vi "concentration percent.vi"(10 "Type Conentration":enum32{"Item 0", "Item 1"}(radio), 11 "Concentration In":T1) -> (3 "Concentration Out":T1)   [LabVIEW 2023]
uses:
  control/Concentrations.ctl
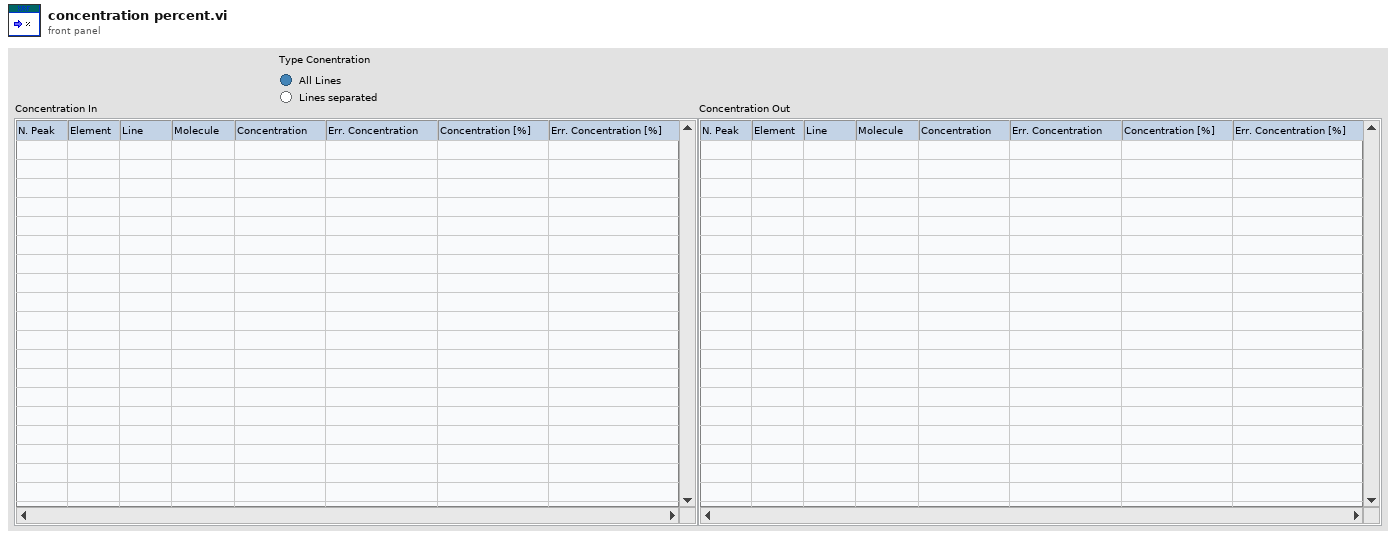
[diagram p1: front panel]
types:
  T1 = typedef "Concentrations.ctl" = string[][]
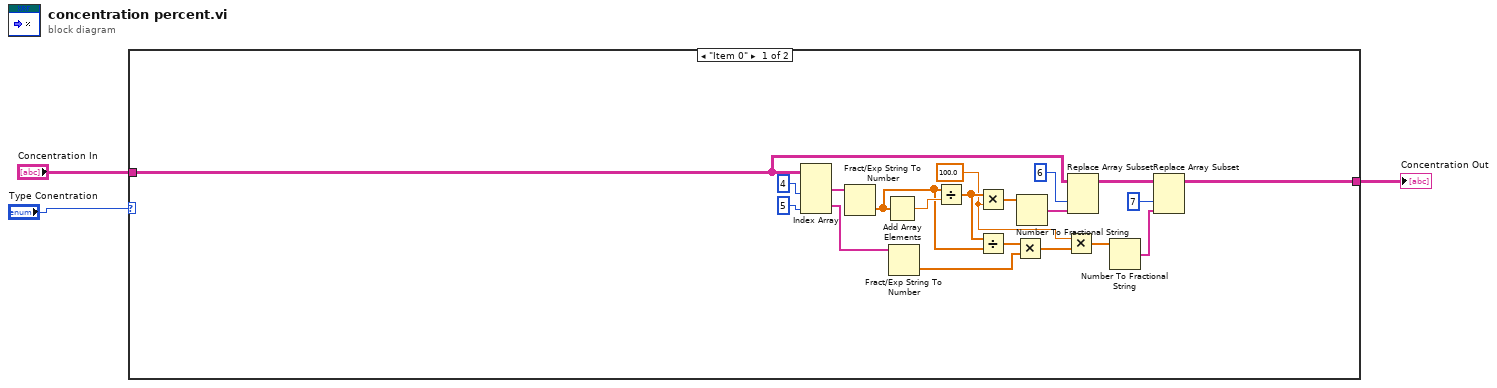
[diagram p0: block diagram]
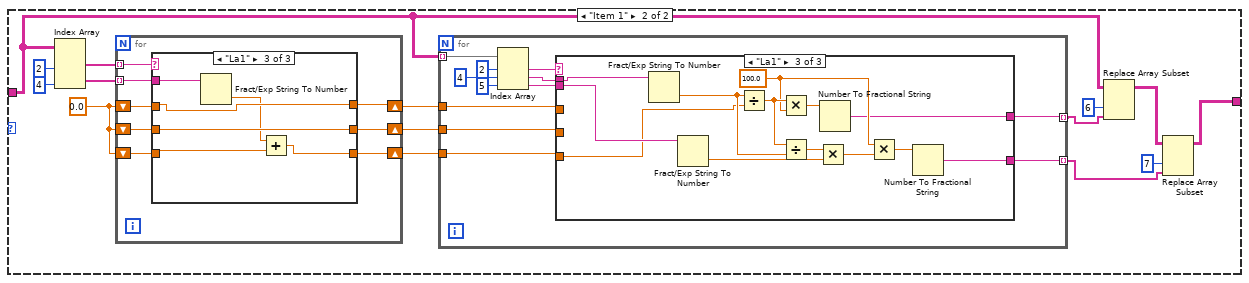
[diagram p2: hidden frame]
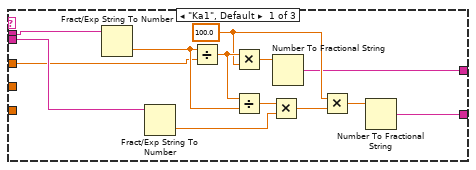
[diagram p3: hidden frame]
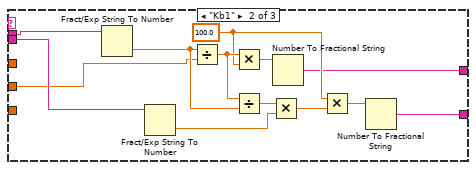
[diagram p4: hidden frame]
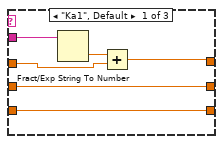
[diagram p5: hidden frame]
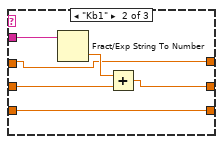
[diagram p6: hidden frame]
diagram:
  n1 = case shown="\"Item 0\"" "Type Conentration" {
    tunnel: [w8 w24] -> w3
    tunnel: "Concentration In" -> [w4 w25]
    frame "Item 0" {
      w7 = 100.0
      n2 = Index Array(array=w4, index (col) #1=4 ("disabled index (col)"), index (col) #2=5 ("index (col)")) -> (element #1=w22:string[], element #2=w16:string[])  [unwired: 2 in]
      n3 = Fract/Exp String To Number(string=w22) -> (number=w14:dbl[])  [unwired: 3 in, 1 out]
      n4 = Add Array Elements(numeric array=w14) -> (sum=w21:dbl)
      n5 = Fract/Exp String To Number(string=w16) -> (number=w13:dbl[])  [unwired: 3 in, 1 out]
      n6 = Divide(x=w14, y=w21) -> (x/y=w12:dbl[])
      n7 = Multiply(x=w12, y=w7) -> (x*y=w20:dbl[])
      n8 = Divide(x=w12, y=w14) -> (x/y=w15:dbl[])
      n9 = Multiply(x=w15, y=w13) -> (x*y=w6:dbl[])
      n10 = Number To Fractional String(number=w20) -> (F-format string=w18:string[])  [unwired: 3 in]
      n11 = Multiply(x=w7, y=w6) -> (x*y=w5:dbl[])
      n12 = Replace Array Subset(array=w4, new element=w18, index (col)=6 ("disabled index (col)")) -> (w11:T1)  [unwired: 1 in]
      n13 = Number To Fractional String(number=w5) -> (F-format string=w9:string[])  [unwired: 3 in]
      n14 = Replace Array Subset(array=w11, new element=w9, index (col)=7 ("disabled index (col)")) -> (w8:T1)  [unwired: 1 in]
    }
    frame "Item 1" {
      w28 = 0.0
      n15 = Index Array(array=w25, index (col) #1=2 ("disabled index (col)"), index (col) #2=4 ("index (col)")) -> (element #1=w35:string[], element #2=w31:string[])  [unwired: 2 in]
      n16 = for {
        tunnel: w35 -> [w97] mode=indexing
        shift-right: [w94] -> w32
        shift-left: w28 -> [w96]
        shift-right: [w93] -> w33
        shift-left: w28 -> [w92]
        shift-right: [w91] -> w34
        shift-left: w28 -> [w90]
        tunnel: w31 -> [w95] mode=indexing
        n17 = case shown="\"La1\"" w97 {
          tunnel: w96 -> [w99 w104 w114]
          tunnel: w95 -> [w103 w109 w115]
          tunnel: [w98 w104 w114] -> w94
          tunnel: [w102 w105 w113] -> w93
          tunnel: w92 -> [w102 w106 w113]
          tunnel: [w101 w108 w112] -> w91
          tunnel: w90 -> [w101 w108 w111]
          frame "Ka1", Default {
            n18 = Fract/Exp String To Number(string=w103) -> (number=w100:dbl)  [unwired: 3 in, 1 out]
            n19 = Add(x=w100, y=w99) -> (x+y=w98:dbl)
          }
          frame "Kb1" {
            n20 = Fract/Exp String To Number(string=w109) -> (number=w107:dbl)  [unwired: 3 in, 1 out]
            n21 = Add(x=w107, y=w106) -> (x+y=w105:dbl)
          }
          frame "La1" {
            n22 = Fract/Exp String To Number(string=w115) -> (number=w110:dbl)  [unwired: 3 in, 1 out]
            n23 = Add(x=w110, y=w111) -> (x+y=w112:dbl)
          }
        }
      }
      n24 = for {
        tunnel: w32 -> [w47]
        tunnel: w33 -> [w46]
        tunnel: w34 -> [w45]
        tunnel: w25 -> [w50] mode=indexing
        tunnel: [w40] -> w37 mode=indexing
        tunnel: [w39] -> w36 mode=indexing
        n25 = Index Array(array=w50, index #1=2 ("index"), index #2=4 ("index"), index #3=5 ("index")) -> (element #1=w48:string, element #2=w42:string, element #3=w41:string)
        n26 = case shown="\"La1\"" w48 {
          tunnel: w47 -> [w53 _ _]
          tunnel: w46 -> [_ w64 _]
          tunnel: w45 -> [_ _ w77]
          tunnel: w42 -> [w55 w68 w81]
          tunnel: w41 -> [w54 w67 w80]
          tunnel: [w52 w66 w79] -> w40
          tunnel: [w51 w65 w78] -> w39
          frame "Ka1", Default {
            w56 = 100.0
            n27 = Fract/Exp String To Number(string=w55) -> (number=w61:dbl)  [unwired: 3 in, 1 out]
            n28 = Fract/Exp String To Number(string=w54) -> (number=w60:dbl)  [unwired: 3 in, 1 out]
            n29 = Divide(x=w61, y=w53) -> (x/y=w59:dbl)
            n30 = Multiply(x=w59, y=w56) -> (x*y=w63:dbl)
            n31 = Divide(x=w59, y=w61) -> (x/y=w62:dbl)
            n32 = Multiply(x=w62, y=w60) -> (x*y=w58:dbl)
            n33 = Number To Fractional String(number=w63) -> (F-format string=w52:string)  [unwired: 3 in]
            n34 = Multiply(x=w56, y=w58) -> (x*y=w57:dbl)
            n35 = Number To Fractional String(number=w57) -> (F-format string=w51:string)  [unwired: 3 in]
          }
          frame "Kb1" {
            w69 = 100.0
            n36 = Fract/Exp String To Number(string=w68) -> (number=w74:dbl)  [unwired: 3 in, 1 out]
            n37 = Fract/Exp String To Number(string=w67) -> (number=w73:dbl)  [unwired: 3 in, 1 out]
            n38 = Divide(x=w74, y=w64) -> (x/y=w72:dbl)
            n39 = Multiply(x=w72, y=w69) -> (x*y=w76:dbl)
            n40 = Divide(x=w72, y=w74) -> (x/y=w75:dbl)
            n41 = Multiply(x=w75, y=w73) -> (x*y=w71:dbl)
            n42 = Number To Fractional String(number=w76) -> (F-format string=w66:string)  [unwired: 3 in]
            n43 = Multiply(x=w69, y=w71) -> (x*y=w70:dbl)
            n44 = Number To Fractional String(number=w70) -> (F-format string=w65:string)  [unwired: 3 in]
          }
          frame "La1" {
            w82 = 100.0
            n45 = Fract/Exp String To Number(string=w81) -> (number=w87:dbl)  [unwired: 3 in, 1 out]
            n46 = Fract/Exp String To Number(string=w80) -> (number=w86:dbl)  [unwired: 3 in, 1 out]
            n47 = Divide(x=w87, y=w77) -> (x/y=w85:dbl)
            n48 = Multiply(x=w85, y=w82) -> (x*y=w89:dbl)
            n49 = Divide(x=w85, y=w87) -> (x/y=w88:dbl)
            n50 = Multiply(x=w88, y=w86) -> (x*y=w84:dbl)
            n51 = Number To Fractional String(number=w89) -> (F-format string=w79:string)  [unwired: 3 in]
            n52 = Multiply(x=w82, y=w84) -> (x*y=w83:dbl)
            n53 = Number To Fractional String(number=w83) -> (F-format string=w78:string)  [unwired: 3 in]
          }
        }
      }
      n54 = Replace Array Subset(array=w25, new element=w37, index (col)=6) -> (w38:T1)  [unwired: 1 in]
      n55 = Replace Array Subset(array=w38, new element=w36, index (col)=7) -> (w24:T1)  [unwired: 1 in]
    }
  }
  "Concentration Out" <- w3
